vi "Visible Control References.vi"(8 "error in":errorcluster, 10 "Visible?":bool, 11 "Control Refs":refnum<vi>[](array[refnum])) -> (0 "error out":errorcluster)   [LabVIEW 2015, in "Diagnostics Addon System Explorer.lvlib"]
uses:
  Diagnostics Addon System Explorer.lvlib
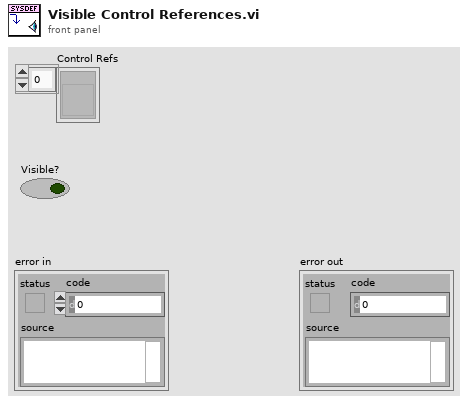
[diagram p1: front panel]
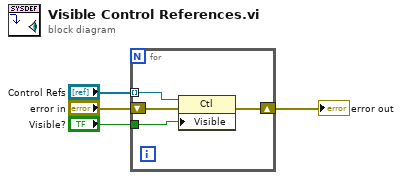
[diagram p0: block diagram]
diagram:
  n1 = for {
    tunnel: "Control Refs" -> [w8] mode=indexing
    tunnel: "Visible?" -> [w7]
    shift-right: [w6] -> w1
    shift-left: "error in" -> [w5]
    n2 = property class="Ctl"(reference=w8, error in=w5, "Visible"=w7) -> (error out=w6:errorcluster)  [unwired: 1 out]
  }
  "error out" <- w1
